vi "Smoothing.vi"(8 "polynomial order":i32=3, 9 "side points":i32=13, 11 "SubtractedSignal":dbl[](array[numeric])) -> (2 "SubSmoothSignal":dbl[](graph))   [LabVIEW 2014]
uses:
  <vilib>/Analysis/3filter.llb/Savitzky-Golay Filter (DBL).vi
  <vilib>/Analysis/NI_AALBase.lvlib
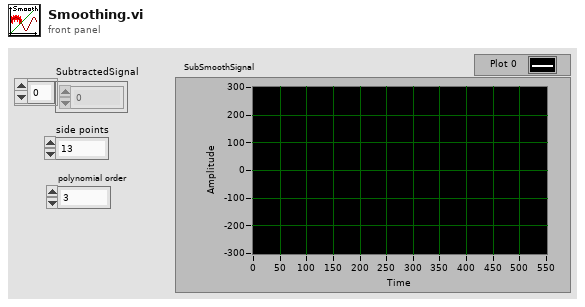
[diagram p1: front panel]
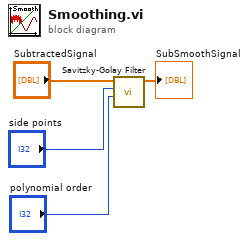
[diagram p0: block diagram]
diagram:
  n1 = call-poly <vilib>:"Savitzky-Golay Filter.vi"("polynomial order"="polynomial order", "side points"="side points", "X"="SubtractedSignal") -> ("Filtered X"=→"SubSmoothSignal":dbl[])  [unwired: 7 in, 1 out]
